vi "Turn to Angle.vi"(6 "PID gains":T1={"proportional gain (Kc)"=1.0, "integral time (Ti, min)"=0.01, "derivative time (Td, min)"=0.0}, 9 "PID?":bool, 10 "Turn now?":bool, 11 "Target Angle":dbl) -> (2 "output":dbl)   [LabVIEW 2016]
uses:
  <vilib>/addons/control/pid/pid.llb/PID (DBL).vi
  <vilib>/addons/control/pid/NI_PID_pid.lvlib
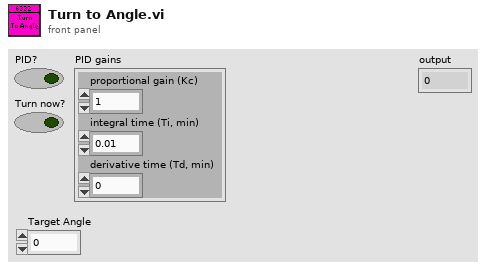
[diagram p1: front panel]
types:
  T1 = cluster{"proportional gain (Kc)":dbl, "integral time (Ti, min)":dbl, "derivative time (Td, min)":dbl}
  T2 = typedef "WPI_GyroDevRef.ctl" = cluster{"DevStatus":errorcluster, "Analog Channel":T3, "Offset":dbl, "Gain (VoltsPerDegree/Second)":dbl, "Gyro Type":enum16{"Analog", "XRS450"}, "Handle":i32, "SPI Bus":T4, "Device Found":bool, "Sample Rate":dbl, "Calibrate On Open":bool}
  T3 = typedef "FPGA_AIChannel.ctl" = enum8{"AI 0", "AI 1", "AI 2", "AI 3", "AI MXP 0", "AI MXP 1", "AI MXP 2", "AI MXP 3", "Invalid"}
  T4 = typedef "spi_bus.ctl" = enum16{"SPI On-Board, CS0", "SPI On-Board, CS1", "SPI On-Board, CS2", "SPI On-Board, CS3", "SPI MXP", "Invalid"}
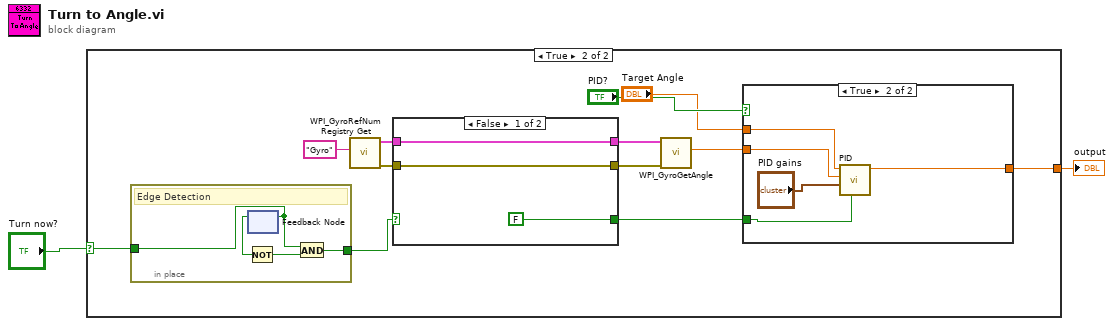
[diagram p0: block diagram]
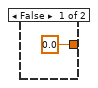
[diagram p2: hidden frame]
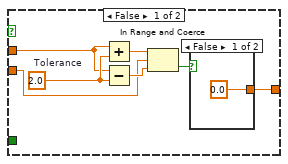
[diagram p3: hidden frame]
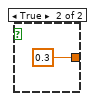
[diagram p4: hidden frame]
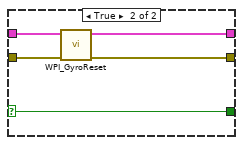
[diagram p5: hidden frame]
diagram:
  n1 = case shown="True" "Turn now?" {
    selector: "Turn now?" -> [_ w13]
    tunnel: [0.0 ("output") w4] -> w1
    frame False {
    }
    frame True {
      n2 = in-place {
        in-place-border: w13 -> [w41]
        in-place-border: [w38] -> w11
        # "Edge Detection"
        n3 = feedback #1() -> (w39:bool)  [unwired: 1 in]
        n4 = Not(x=w39) -> (.not. x?=w40:bool)
        n5 = feedback-in #1(w41) -> ()
        n6 = And(x=w41, y=w40) -> (x .and. y?=w38:bool)
      }
      n7 = call <vilib>:"WPI_GyroRefNum Registry Get.vi"("refnum name"="Gyro") -> ("error out"=w9:errorcluster, "GyroDevRef"=w10:T2)  [unwired: 9 in]
      n8 = case shown="False" w11 {
        selector: w11 -> [_ w33]
        tunnel: [w31 w37] -> w15
        tunnel: [w32 w36] -> w14
        tunnel: w10 -> [w32 w35]
        tunnel: w9 -> [w31 w34]
        tunnel: [FALSE w33] -> w7
        frame False {
        }
        frame True {
          n9 = call <vilib>:"WPI_GyroReset.vi"("error in"=w34, "GyroDevRef"=w35) -> ("error out"=w37:errorcluster, "GyroDevRef"=w36:T2)  [unwired: 8 in]
        }
      }
      n10 = call <vilib>:"WPI_GyroGetAngle.vi"("error in"=w15, "GyroDevRef"=w14) -> ("Angle"=w8:dbl)  [unwired: 5 in, 4 out]
      n11 = case shown="True" "PID?" {
        tunnel: w8 -> [w16 w29]
        tunnel: w7 -> [_ w28]
        tunnel: "Target Angle" -> [w19 w27]
        tunnel: [w17 w26] -> w4
        frame False {
          w21 = 2.0  # Tolerance
          n12 = Add(x=w19, y=w21) -> (x+y=w20:dbl)
          n13 = Subtract(x=w19, y=w21) -> (x-y=w22:dbl)
          n14 = In Range and Coerce(upper limit=w20, x=w16, lower limit=w22) -> (In Range?=w18:bool)  [unwired: 1 out]
          n15 = case shown="False" w18 {
            tunnel: [0.0 0.3] -> w17
            frame False {
            }
            frame True {
            }
          }
        }
        frame True {
          n16 = call-poly <vilib>:"PID.vi"("reinitialize? (F)"=w28, "PID gains"="PID gains", "process variable"=w29, "setpoint"=w27) -> ("output"=w26:dbl)  [unwired: 6 in, 1 out]
        }
      }
    }
  }
  "output" <- w1
